vi "Create Datafile Entry.vi"(0 "Serial Number":u32=1, 1 "Resistance 1":dbl=nan, 2 "STD 1":dbl=nan, 3 "File Name":path=path "C:/Users/qmgmit/Desktop/default_datafile.txt", 4 "Phase 1":dbl=nan, 5 "Start time":timestamp=timestamp(3753394826.5765777 s since 1904-01-01), 6 "Phase 2":dbl=nan, 7 "Temperature":dbl=300.0, 9 "Field":dbl=200.0, 11 "Theta":dbl, 12 "Resistance 2":dbl=nan, 13 "STD 2":dbl=nan, 14 "Current Level":dbl=1e-05) -> (15 "Datapoint Array":dbl[](array[numeric]))   [LabVIEW 2020]
uses:
  <vilib>/Utility/file.llb/Write Delimited Spreadsheet (string).vi
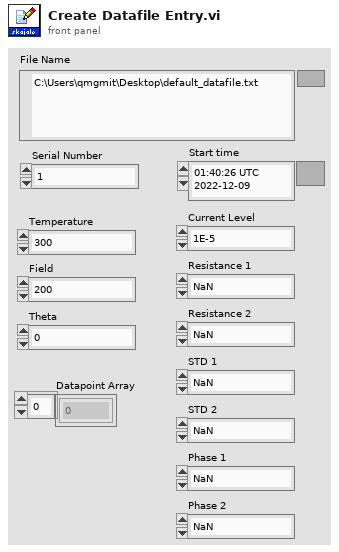
[diagram p1: front panel]
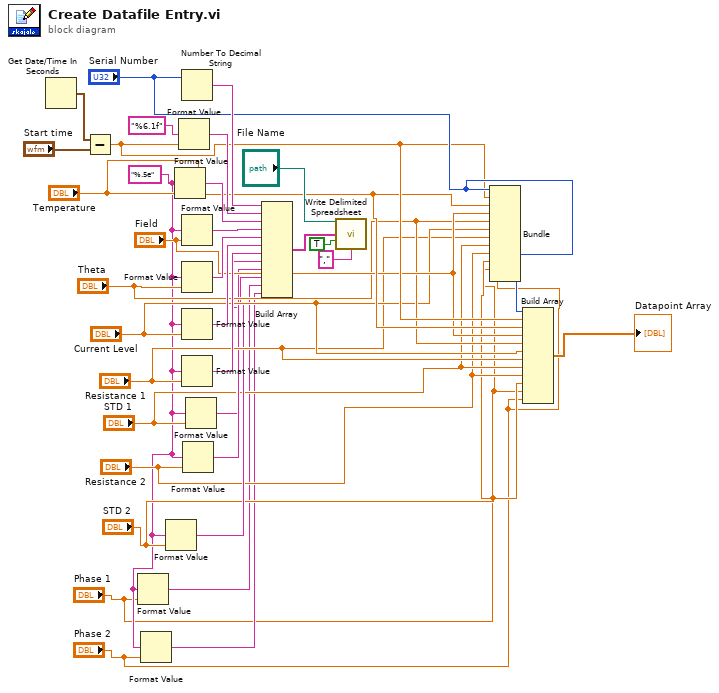
[diagram p0: block diagram]
diagram:
  w5 = "%.5e" ("format string")
  n1 = Get Date/Time In Seconds() -> (seconds since 1Jan1904=w29:timestamp)
  n2 = Subtract(x=w29, y="Start time") -> (x-y=w19:dbl)
  n3 = Format Value(format string=w5, value (0)="Phase 1") -> (output string=w4:string)  [unwired: 1 in]
  n4 = Format Value(format string=w5, value (0)="Phase 2") -> (output string=w3:string)  [unwired: 1 in]
  n5 = Format Value(format string=w5, value (0)="STD 2") -> (output string=w10:string)  [unwired: 1 in]
  n6 = Format Value(format string=w5, value (0)="Temperature") -> (output string=w25:string)  [unwired: 1 in]
  n7 = Format Value(format string="%6.1f", value (0)=w19) -> (output string=w26:string)  [unwired: 1 in]
  n8 = Number To Decimal String(number="Serial Number") -> (decimal integer string=w30:string)  [unwired: 1 in]
  n9 = Format Value(format string=w5, value (0)="Field") -> (output string=w24:string)  [unwired: 1 in]
  n10 = Format Value(format string=w5, value (0)="Theta") -> (output string=w23:string)  [unwired: 1 in]
  n11 = Format Value(format string=w5, value (0)="Current Level") -> (output string=w22:string)  [unwired: 1 in]
  n12 = Format Value(format string=w5, value (0)="Resistance 1") -> (output string=w21:string)  [unwired: 1 in]
  n13 = Format Value(format string=w5, value (0)="Resistance 2") -> (output string=w12:string)  [unwired: 1 in]
  n14 = Format Value(format string=w5, value (0)="STD 1") -> (output string=w11:string)  [unwired: 1 in]
  n15 = Build Array(w30, w26, w25, w24, w23, w22, w21, w11, w12, w10, w4, w3) -> (w32:string[])
  n16 = call-poly <vilib>:"Write Delimited Spreadsheet.vi"("file path (dialog if empty)"="File Name", "1D data"=w32, "append to file? (new file:F)"=TRUE, "delimiter (\\t)"="," ("delimiter (\\t)")) -> ()  [unwired: 10 in, 2 out]
  n17 = Bundle("Serial Number"="Serial Number", w19, "Temperature"="Temperature", "Field"="Field", "Theta"="Theta", "Current Level"="Current Level", "Resistance 1"="Resistance 1", "STD 1"="STD 1", "Resistance 2"="Resistance 2", "STD 2"="STD 2", "Phase 1"="Phase 1", "Phase 2"="Phase 2") -> ()  [unwired: 1 in, 1 out]
  n18 = Build Array("Serial Number", w19, "Temperature", "Field", "Theta", "Current Level", "Resistance 1", "STD 1", "Resistance 2", "STD 2", "Phase 1", "Phase 2") -> (→"Datapoint Array":dbl[])
